vi "pessimize_objective.vi"(9 "Find gradient":bool, 10 "data":T1, 11 "X":dbl[](array[numeric]) format="%#_3p") -> (0 "error out":errorcluster, 2 "Gradient":dbl[](array[numeric]) format="%#_3p", 3 "f(X)":dbl)   [LabVIEW 2013]
uses:
  <vilib>/gmath/NumericalOptimization/objective function data.ctl
  pessimize_objective_fun_info.ctl
  calibration/point_selector.ctl
  ui_override_opts.ctl
  <vilib>/gmath/NI_Gmath.lvlib
panel:
  # "Compute gradient"
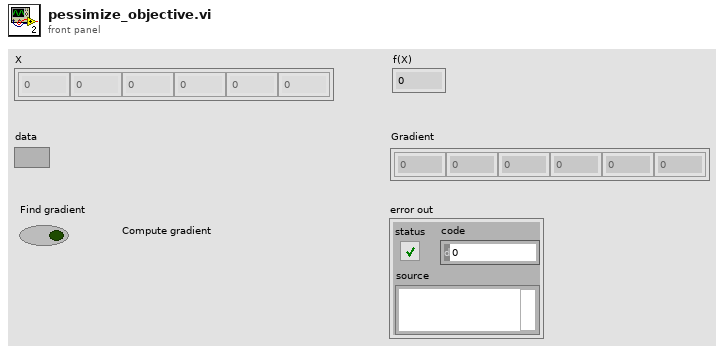
[diagram p1: front panel]
types:
  T1 = typedef "NI_Gmath.lvlib/objective function data.ctl" = variant
  T2 = typedef "pessimize_objective_fun_info.ctl" = cluster{"Error criterion":enum16{"Translation", "Orientation", "Moment"}, "Scale factors":dbl[], "Gradient increment":dbl[], "Pose bias":dbl[], "Extra end transform":dbl[], "Point selector":T3, "Trace length":dbl, "Override in":T4, "Optimization status":refnum<vi>, "stop":refnum<vi>}
  T3 = typedef "point_selector.ctl" = cluster{"Pose mode":enum16{"Light", "Handle", "Output"}, "Light number":i32}
  T4 = typedef "ui_override_opts.ctl" = cluster{"Triggering":bool, "Parameters":bool, "Stimulus":bool, "Calibration":bool, "Modes":bool}
  T5 = typedef "NI_Matrix.lvlib/RealMatrix.ctl" = dbl[][]
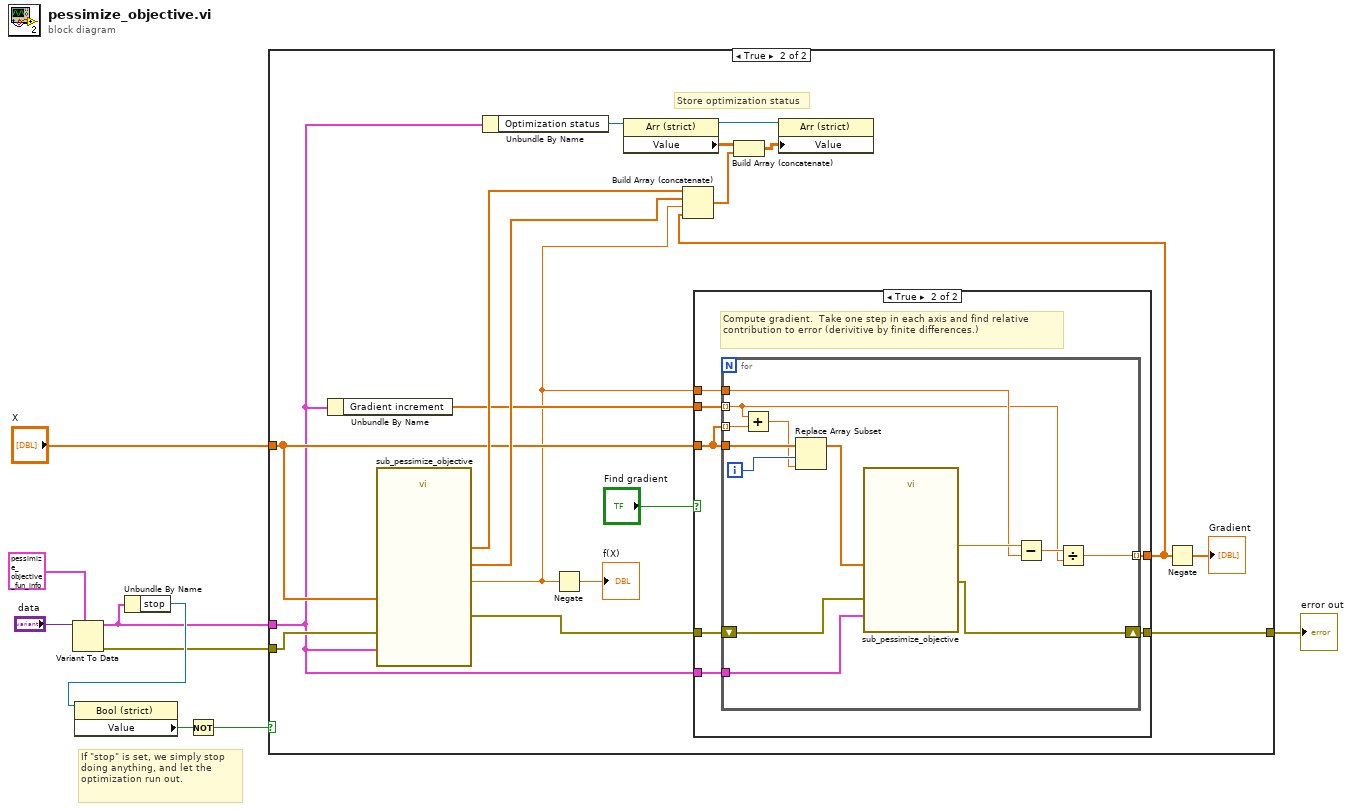
[diagram p0: block diagram]
diagram:
  # "If \"stop\" is set, we simply stop doing anything, and let the optimization run out."
  n1 = Variant To Data(type=T2 {"Error criterion"=enum."Translation", "Scale factors"=[], "Gradient increment"=[], "Pose bias"=[], "Extra end transform"=[], "Point selector"={"Pose mode"=enum."Light", "Light number"=0}, "Trace length"=0.0, "Override in"={"Triggering"=FALSE, "Parameters"=FALSE, "Stimulus"=FALSE, "Calibration"=FALSE, "Modes"=FALSE}, "Optimization status"=refnum, "stop"=refnum} ("Pessimize fun info"), Variant="data") -> (data=w6:T2, error out=w5:errorcluster)  [unwired: 1 in]
  n2 = Unbundle By Name(w6) -> ("stop"=w7:refnum<vi>)
  n3 = property class="Bool (strict)"(reference=w7) -> ("Value"=w8:bool)  [unwired: 1 in, 2 out]
  n4 = Not(x=w8) -> (.not. x?=w9:bool)
  n5 = case shown="True" w9 {
    tunnel: "X" -> [_ w17]
    tunnel: [_ w13] -> w2
    tunnel: w6 -> [_ w14]
    tunnel: w5 -> [_ w27]
    frame False {
    }
    frame True {
      # "Store optimization status"
      n6 = Unbundle By Name(w14) -> ("Gradient increment"=w18:dbl[])
      n7 = call "sub_pessimize_objective.vi"("error in"=w27, "Pessimize fun info"=w14, "X"=w17) -> ("error out"=w15:errorcluster, "f(X)"=w10:dbl, "Error vector"=w26:dbl[], "Pose command"=w20:dbl[])  [unwired: 5 in]
      n8 = Unbundle By Name(w14) -> ("Optimization status"=w25:refnum<vi>)
      n9 = Negate(x=w10) -> (-x=→"f(X)":dbl)
      n10 = property class="Arr (strict)"(reference=w25) -> (reference out=w21:refnum<vi>, "Value"=w24:T5)  [unwired: 1 in, 1 out]
      n11 = case shown="True" "Find gradient" {
        tunnel: w18 -> [_ w35]
        tunnel: w17 -> [_ w34]
        tunnel: w15 -> [w28 w33]
        tunnel: w14 -> [_ w32]
        tunnel: w10 -> [_ w31]
        tunnel: [_ w30] -> w11
        tunnel: [w28 w29] -> w13
        frame False {
          # "Not computing gradient"
        }
        frame True {
          # "Compute gradient.  Take one step in each axis and find relative contribution to error (derivitive by finite differences.)"
          n12 = for {
            tunnel: w35 -> [w37] mode=indexing
            tunnel: w34 -> [w48]
            tunnel: w34 -> [w46] mode=indexing
            shift-right: [w42] -> w29
            shift-left: w33 -> [w43]
            tunnel: w32 -> [w41]
            tunnel: w31 -> [w39]
            tunnel: [w36] -> w30 mode=indexing
            i -> [w47]
            n13 = Add(x=w37, y=w46) -> (x+y=w45:dbl)
            n14 = Replace Array Subset(array=w48, new element=w45, index=w47) -> (w44:dbl[])
            n15 = call "sub_pessimize_objective.vi"("error in"=w43, "Pessimize fun info"=w41, "X"=w44) -> ("error out"=w42:errorcluster, "f(X)"=w40:dbl)  [unwired: 5 in, 2 out]
            n16 = Subtract(x=w40, y=w39) -> (x-y=w38:dbl)
            n17 = Divide(x=w38, y=w37) -> (x/y=w36:dbl)
          }
        }
      }
      n18 = Build Array (concatenate)(w20, w26, w10, w11) -> (w23:dbl[])
      n19 = Build Array (concatenate)(w24, w23) -> (w22:T5)
      n20 = property class="Arr (strict)"(reference=w21, "Value"=w22) -> ()  [unwired: 1 in, 2 out]
      n21 = Negate(x=w11) -> (-x=→"Gradient":dbl[])
    }
  }
  "error out" <- w2
